vi "Propagation.vi"() -> ()   [LabVIEW 2020]
uses:
  StatisticsData.ctl
  HasoSlopes.lvclass
  Pupil.lvclass
  ComputePhaseSet.lvclass
  WavefrontReconstructionMode.ctl
  Phase.lvclass
  HasoField.lvclass
  SurfaceFloat.lvclass
  General dimensions definition.ctl
  Point2D.ctl
  Point2Df.ctl
  HasoData.lvclass
panel:
  out "PSF values":sgl[][](graph)
  in  "Slopes file name":string="Data\\data_phase_computation.has"
  in  "Haso configuration file name":string="Data\\config_file_haso.dat"
  out "PSF Statistics":T1
  out "error out":errorcluster
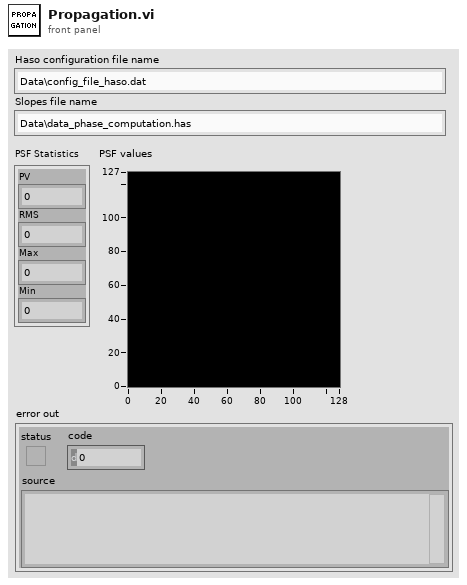
[diagram p1: front panel]
types:
  T1 = typedef "StatisticsData.ctl" = cluster{"PV":sgl, "RMS":dbl, "Max":sgl, "Min":sgl}
  T2 = typedef "General dimensions definition.ctl" = cluster{"Size":T3, "Step":T4}
  T3 = typedef "Point2D.ctl" = cluster{"X":u32, "Y":u32}
  T4 = typedef "Point2Df.ctl" = cluster{"X":sgl, "Y":sgl}
  T5 = cluster{"null_phase":bool, "flat_intensity":bool}
  T6 = typedef "WavefrontReconstructionMode.ctl" = enum16{"None", "Modal_Legendre", "Modal_Zernike", "Zonal", "Modal_Zonal_Zernike", "Modal_Zonal_Legendre"}
  T7 = typedef "DataHaso acquisition information.ctl" = cluster{"HASO information":T8, "Acquisition information":T9, "SLOPES ENGINE information":T13, "Source wavelength (nm)":dbl, "FillPercent_%":dbl, "session_name":string}
  T8 = typedef "HASO information.ctl" = cluster{"HASO serial number":string, "HASO model":string, "Lower calibration wavelength (nm)":dbl, "Upper calibration wavelength (nm)":dbl, "Revision":i32}
  T9 = typedef "Image information.ctl" = cluster{"Image general information":T10, "Acquisition information":T11, "Number of pixels":T3, "Number of bits":T12}
  T10 = typedef "Image general information.ctl" = cluster{"Camera serial number":string, "Smearing removed":bool, "Background image removed":bool, "Time Stamp":timestamp, "Comment":string, "Camera_MAX_Level":i32}
  T11 = typedef "Image acquisition information.ctl" = cluster{"Exposure duration (us)":i32, "Exposure duration specified (us)":i32, "Gain":sgl, "Number of summed images":i32, "Trigger type":string}
  T12 = typedef "Data alignment enum.ctl" = enum16{"8", "16", "32"}
  T13 = typedef "SlopesEngineSetup.ctl" = cluster{"Start sub-aperture":T3, "Pupil average":dbl, "AutoStartSub-aperture":bool}
  T14 = cluster{"tiltX_mrad":sgl, "tiltY_mrad":dbl, "radius_mm":sgl, "focus_Xpos_mm":sgl, "focus_Ypos_mm":sgl, "astig_angle_rad":sgl, "sagittal_focal_length_mm":sgl, "tangential_focal_length_mm":sgl}
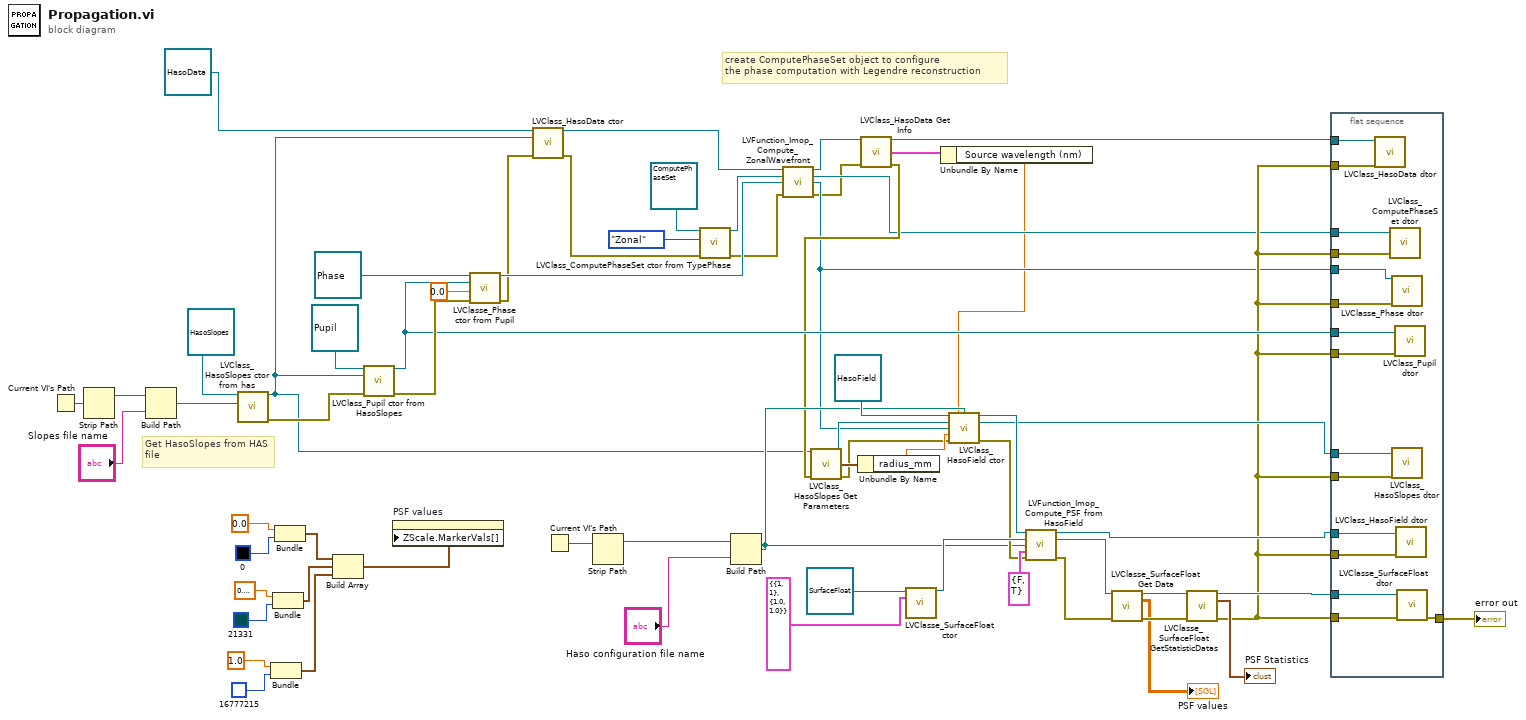
[diagram p0: block diagram]
diagram:
  # "create ComputePhaseSet object to configure\nthe phase computation with Legendre reconstruction"
  # "Get HasoSlopes from HAS file"
  n1 = Current VI's Path() -> (path=w41:path)
  n2 = Strip Path(path=w41) -> (stripped path=w35:path)  [unwired: 1 out]
  n3 = Build Path(base path=w35, name or relative path="Slopes file name") -> (appended path=w8:path)
  n4 = call "LVClass_HasoSlopes ctor from has.vi"("HasoSlopes (const)"=refnum<class "HasoSlopes.lvclass"> refnum ("HasoSlopes in"), ".has path"=w8) -> ("HasoSlopes (new)"=w14:refnum<class "HasoSlopes.lvclass">, "error out"=w51:errorcluster)  [unwired: 12 in]
  n5 = Bundle(sgl 1.0, u32 16777215) -> (w17:cluster{sgl, u32})  [unwired: 1 in]
  n6 = Bundle(sgl 0.2, u32 21331) -> (w16:cluster{sgl, u32})  [unwired: 1 in]
  n7 = Bundle(0.0, u32 0) -> (w21:cluster{dbl, u32})  [unwired: 1 in]
  n8 = Build Array(w21, w16, w17) -> (w20:cluster{dbl, u32}[])
  n9 = call "LVClass_Pupil ctor from HasoSlopes.vi"("Pupil (const)"=refnum<class "Pupil.lvclass"> refnum ("Pupil in"), "HasoSlopes"=w14, "error in (no error)"=w51) -> ("Pupil (new)"=w48:refnum<class "Pupil.lvclass">, "error out"=w60:errorcluster)  [unwired: 10 in, 1 out]
  n10 = property on="PSF values" class="IntGraph (strict)"("ZScale.MarkerVals[]"=w20) -> ()  [unwired: 2 in, 2 out]
  n11 = call "LVClasse_Phase ctor from Pupil.vi"("Phase (const)"=refnum<class "Phase.lvclass"> refnum ("Phase in"), "Pupil"=w48, "coef"=sgl 0.0, "error in (no error)"=w60) -> ("Phase (new)"=w12:refnum<class "Phase.lvclass">, "error out"=w4:errorcluster)  [unwired: 9 in, 1 out]
  n12 = call "LVClass_HasoData ctor.vi"("HasoData (const)"=refnum<class "HasoData.lvclass"> refnum ("HasoData in"), "HasoSlopes"=w14, "error in (no error)"=w4) -> ("HasoData (new)"=w5:refnum<class "HasoData.lvclass">, "error out"=w3:errorcluster)  [unwired: 10 in, 1 out]
  n13 = Current VI's Path() -> (path=w38:path)
  n14 = Strip Path(path=w38) -> (stripped path=w36:path)  [unwired: 1 out]
  n15 = call "LVClass_ComputePhaseSet ctor from TypePhase.vi"("ComputePhaseSet (const)"=refnum<class "ComputePhaseSet.lvclass"> refnum ("ComputePhaseSet in"), "TypePhase"=WavefrontReconstructionMode."Zonal", "error in (no error)"=w3) -> ("ComputePhaseSet (new)"=w13:refnum<class "ComputePhaseSet.lvclass">, "error out"=w2:errorcluster)  [unwired: 11 in]
  n16 = Build Path(base path=w36, name or relative path="Haso configuration file name") -> (appended path=w37:path)
  n17 = call "LVFunction_Imop_Compute_ZonalWavefront.vi"("HasoData.lvclass"=w5, "ComputePhaseSet.lvclass"=w13, "Phase"=w12, "error constant"=w2) -> ("HasoData.lvclass (dup)"=w11:refnum<class "HasoData.lvclass">, "ComputePhaseSet.lvclass 2"=w10:refnum<class "ComputePhaseSet.lvclass">, "Phase"=w9:refnum<class "Phase.lvclass">, "error out"=w1:errorcluster)  [unwired: 8 in]
  n18 = call "LVClass_HasoData Get Info.vi"("HasoData in"=w11, "error in (no error)"=w1) -> ("HasoData out"=w28:refnum<class "HasoData.lvclass">, "DataHaso acquisition information"=w29:T7, "error out"=w15:errorcluster)  [unwired: 11 in]
  n19 = call "LVClass_HasoSlopes Get Parameters.vi"("HasoSlopes in"=w14, "error in (no error)"=w15) -> ("HasoSlopes out"=w50:refnum<class "HasoSlopes.lvclass">, "Pamameter"=w49:T14, "error out"=w27:errorcluster)  [unwired: 11 in]
  n20 = Unbundle By Name(w49) -> ("radius_mm"=w34:sgl)
  n21 = call "LVClasse_SurfaceFloat ctor.vi"("SurfaceFloat (const)"=refnum<class "SurfaceFloat.lvclass"> refnum ("SurfaceFloat in"), "Dimensions_um"=T2 {"Size"={"X"=1, "Y"=1}, "Step"={"X"=1.0, "Y"=1.0}} ("Dimensions_µm")) -> ("SurfaceFloat (new)"=w57:refnum<class "SurfaceFloat.lvclass">)  [unwired: 12 in, 1 out]
  n22 = Unbundle By Name(w29) -> ("Source wavelength (nm)"=w7:dbl)
  n23 = call "LVClass_HasoField ctor.vi"("HasoField (const)"=refnum<class "HasoField.lvclass"> refnum ("HasoField in"), "wavelenght nm"=w7, "haso_config_file_path"=w37, "HasoSlopes"=w50, "Phase"=w9, "radius_of_curvature _ mm"=w34, "error in (no error)"=w27) -> ("HasoField (new)"=w58:refnum<class "HasoField.lvclass">, "HasoSlopes (dup)"=w42:refnum<class "HasoSlopes.lvclass">, "error out"=w43:errorcluster)  [unwired: 4 in, 2 out]
  n24 = call "LVFunction_Imop_Compute_PSF from HasoField.vi"("HasoField in"=w58, "Surface PSF"=w57, "Path"=w37, "param"=T5 {"null_phase"=FALSE, "flat_intensity"=TRUE}, "error in (no error)"=w43) -> ("HasoField out"=w53:refnum<class "HasoField.lvclass">, "Surface PSF"=w33:refnum<class "SurfaceFloat.lvclass">, "error out"=w32:errorcluster)  [unwired: 8 in]
  n25 = call "LVClasse_SurfaceFloat Get Data.vi"("SurfaceFloat in"=w33, "error in (no error)"=w32) -> ("SurfaceFloat out"=w47:refnum<class "SurfaceFloat.lvclass">, "data"=→"PSF values":sgl[][], "error out"=w46:errorcluster)  [unwired: 11 in]
  n26 = call "LVClasse_SurfaceFloat GetStatisticDatas.vi"("SurfaceFloat in"=w47, "error in (no error)"=w46) -> ("SurfaceFloat out"=w44:refnum<class "SurfaceFloat.lvclass">, "StatisticsData"=→"PSF Statistics":T1, "error out"=w31:errorcluster)  [unwired: 11 in]
  n27 = flat-sequence {
    tunnel: w42 -> [w80]
    tunnel: w53 -> [w79]
    tunnel: w44 -> [w78]
    tunnel: w10 -> [w77]
    tunnel: w28 -> [w76]
    tunnel: w48 -> [w75]
    tunnel: w31 -> [w74]
    tunnel: w31 -> [w73]
    tunnel: w31 -> [w72]
    tunnel: w31 -> [w71]
    tunnel: w31 -> [w70]
    tunnel: w31 -> [w69]
    tunnel: w31 -> [w68]
    tunnel: [w67] -> w30
    tunnel: w9 -> [w66]
    frame #0 {
      n28 = call "LVClass_HasoData dtor.vi"("HasoData in"=w76, "error in (no error)"=w69) -> ()  [unwired: 12 in, 2 out]
      n29 = call "LVClass_ComputePhaseSet dtor.vi"("ComputePhaseSet in"=w77, "error in (no error)"=w68) -> ()  [unwired: 12 in, 2 out]
      n30 = call "LVClasse_Phase dtor.vi"("Phase in"=w66, "error in (no error)"=w70) -> ()  [unwired: 12 in, 2 out]
      n31 = call "LVClass_HasoSlopes dtor.vi"("HasoSlopes in"=w80, "error in (no error)"=w72) -> ()  [unwired: 12 in, 2 out]
      n32 = call "LVClass_Pupil dtor.vi"("Pupil in"=w75, "error in (no error)"=w71) -> ()  [unwired: 12 in, 2 out]
      n33 = call "LVClass_HasoField dtor.vi"("HasoField in"=w79, "error in (no error)"=w73) -> ()  [unwired: 12 in, 2 out]
      n34 = call "LVClasse_SurfaceFloat dtor.vi"("SurfaceFloat in"=w78, "error in (no error)"=w74) -> ("error out"=w67:errorcluster)  [unwired: 12 in, 1 out]
    }
  }
  "error out" <- w30
